vi "TCP Engine.vi"(7 "Hardware Info":T1[](array[typedef]) {"Is Present?" items=["Initializing"=-2, "Unknown"=-1, "Not Present"=0, "Present"=1]}, 8 "error in":errorcluster, 10 "Port":u16=6001, 11 "IP Address":string) -> (0 "error out":errorcluster)   [LabVIEW 2024, in "TCP Engine.lvlib"]
doc: "This VI will communicate with HOST through TCP/IP Communication, also it communicates with all engines through queue mechanism.\n\n\n\nAll Rights Reserved © 2023 SyncSols"
uses:
  TCP Engine.lvlib
  Controls/TCP Engine State Machine Data Cluster.ctl
  Controls/TCP Engine Send Loop Data.ctl
  Main Engine/Controls/Main Engine Command Cluster.ctl
  Main Engine/Controls/Main Engine TCP Command Data.ctl
  Main Engine/Controls/Main Engine Hardware Info Data Cluster.ctl
  Controls/TCP Engine Q Driver Options.ctl
  Controls/TCP Engine State Machine Cases.ctl
  Main Engine/Controls/Main Engine Q Option.ctl
  <vilib>/NI_Real-Time Target Support.lvlib
panel:
  out "notifier":refnum<notifier>
  in  "Data Cluster":T2 {"Hardware Info"."Is Present?" items=["Initializing"=-2, "Unknown"=-1, "Not Present"=0, "Present"=1]}
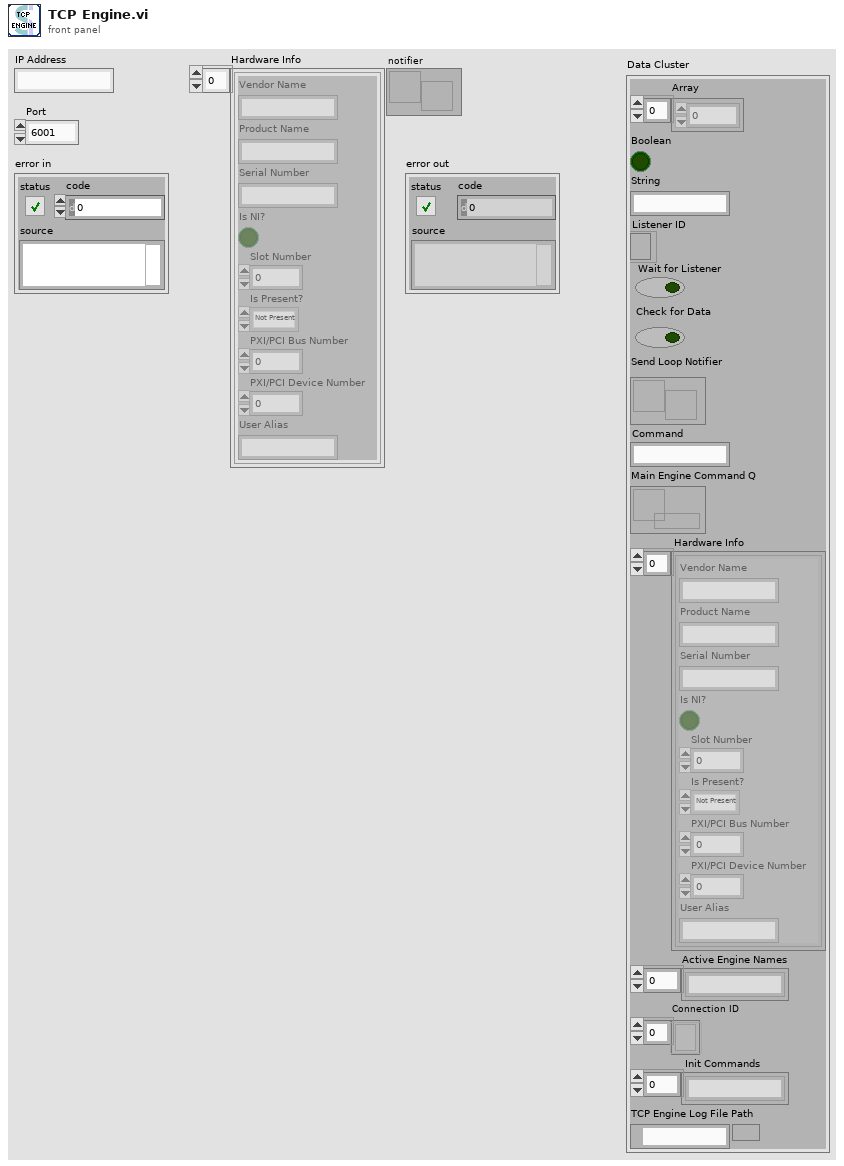
[diagram p1: front panel]
types:
  T1 = typedef "Main Engine Hardware Info Data Cluster.ctl" = cluster{"Vendor Name":string, "Product Name":string, "Serial Number":string, "Is NI?":bool, "Slot Number":i32, "Is Present?":i32, "PXI/PCI Bus Number":u32, "PXI/PCI Device Number":u32, "User Alias":string}
  T2 = typedef "TCP Engine.lvlib/TCP Engine State Machine Data Cluster.ctl" = cluster{"Array":dbl[], "Boolean":bool, "String":string, "Listener ID":refnum<k5>, "Wait for Listener":bool, "Check for Data":bool, "Send Loop Notifier":refnum<notifier>, "Command":string, "Main Engine Command Q":refnum<queue>, "Hardware Info":T1[], "Active Engine Names":string[], "Connection ID":refnum<k5>[], "Init Commands":string[], "TCP Engine Log File Path":path}
  T3 = typedef "TCP Engine.lvlib/TCP Engine Send Loop Data.ctl" = cluster{"Start Send Loop":bool, "Stop Send Loop":bool, "Connection ID":refnum<k5>[], "Log File Path":path}
  T4 = typedef "TCP Engine.lvlib/TCP Engine State Machine Cases.ctl" = enum16{">Poll", ".........State Machine.........", ">Init", ">Init Configuration", ">Decode Configuration", ">Error", ">Exit", "..........TCP Engine..........", ">Wait for Listener", ">Get Msg from HOST", ">Decode the Command", ">Create Listerner ID"}
  T5 = typedef "TCP Engine.lvlib/TCP Engine Q Driver Options.ctl" = enum16{"Initialize", "EnQ", "DeQ", "EnQ at Opp", "Get Q Status", "Flush Q", "Release Q"}
  T6 = typedef "Main Engine Q Option.ctl" = enum16{"Init", "Get"}
  T7 = typedef "Main Engine Command Cluster.ctl" = cluster{"State":T8, "Interface":string, "Engine Name":string, "Varient Data":variant, "SubCmd":string, "Serial Mode":string, "ARINC Board":u8, "Ethernet Mode":u8, "CPU Frequency":dbl}
  T8 = typedef "Main Engine TCP Command Data.ctl" = enum16{"Get HW Info", "Launch Module", "Get CPU Load", "Close CPU Load", "Exit"}
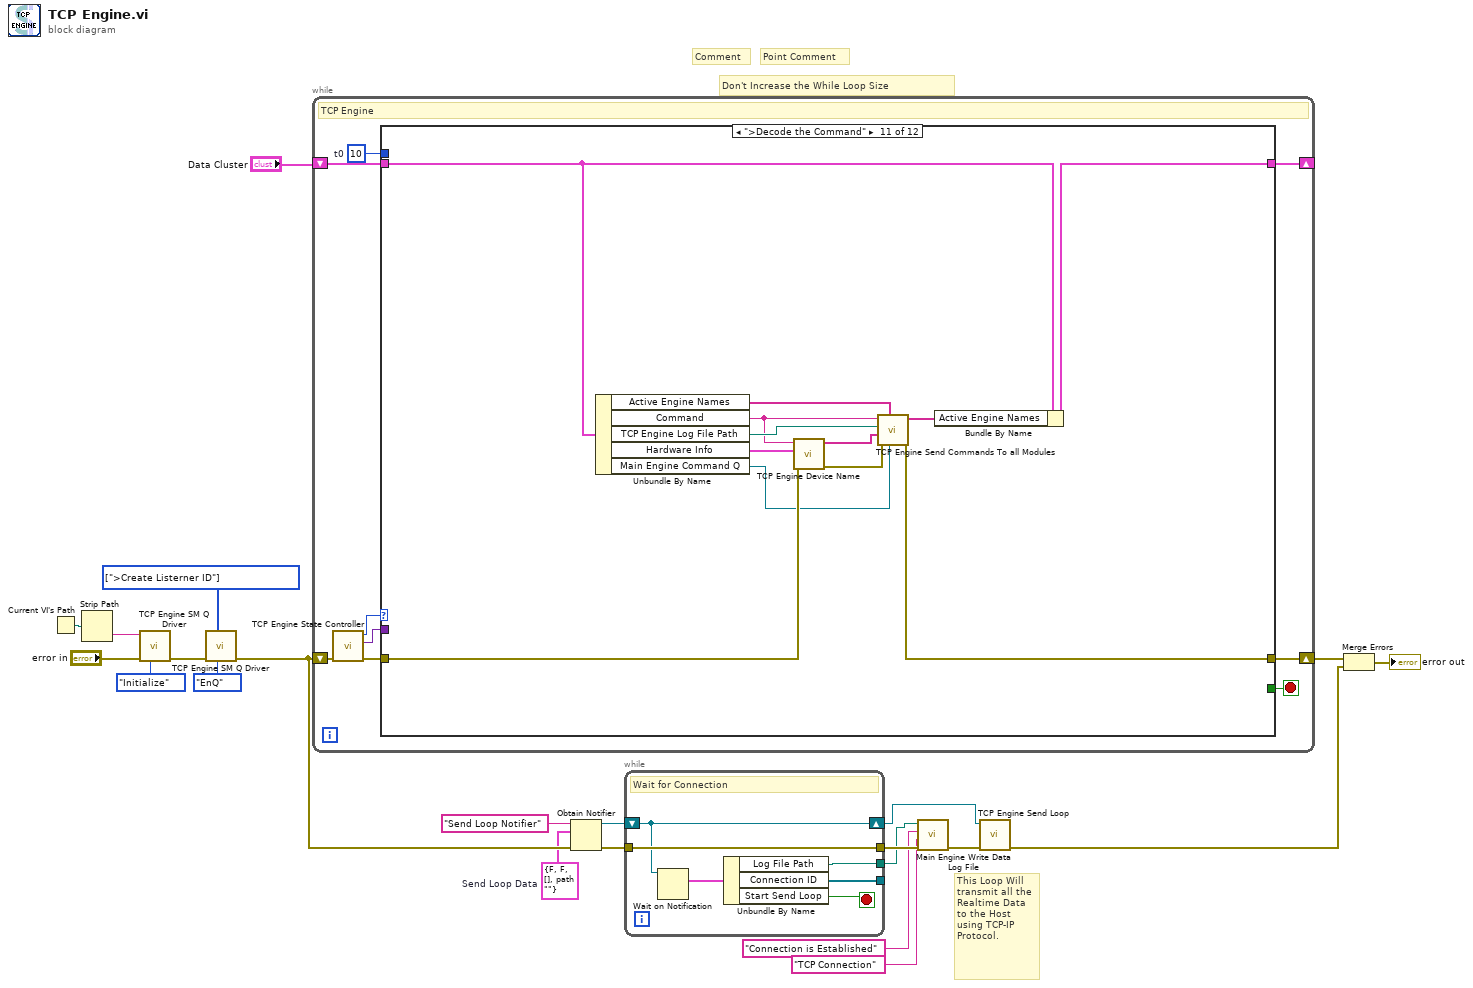
[diagram p0: block diagram]
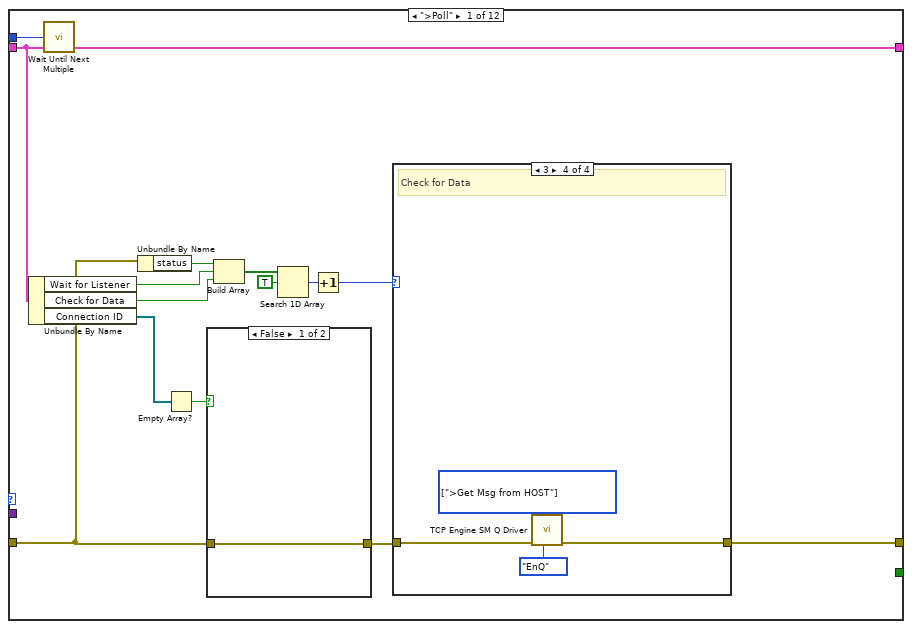
[diagram p2: hidden frame]
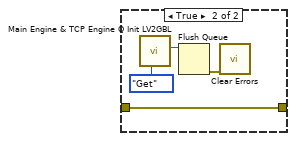
[diagram p3: hidden frame]
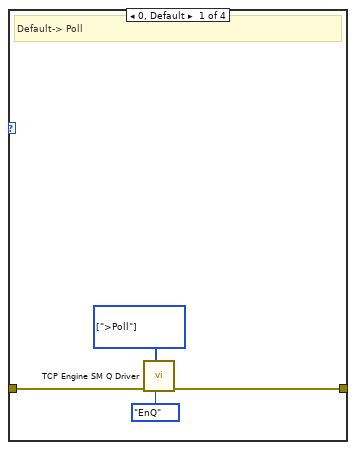
[diagram p4: hidden frame]
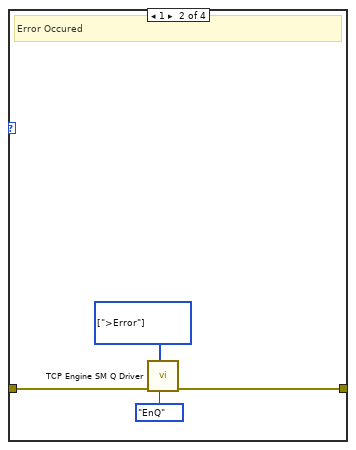
[diagram p5: hidden frame]
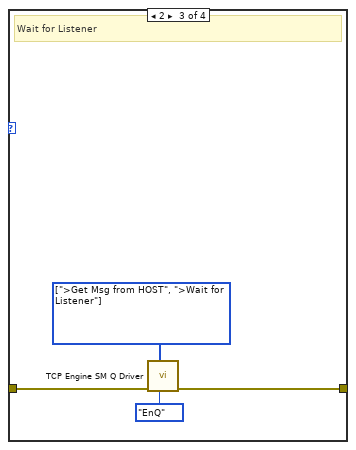
[diagram p6: hidden frame]
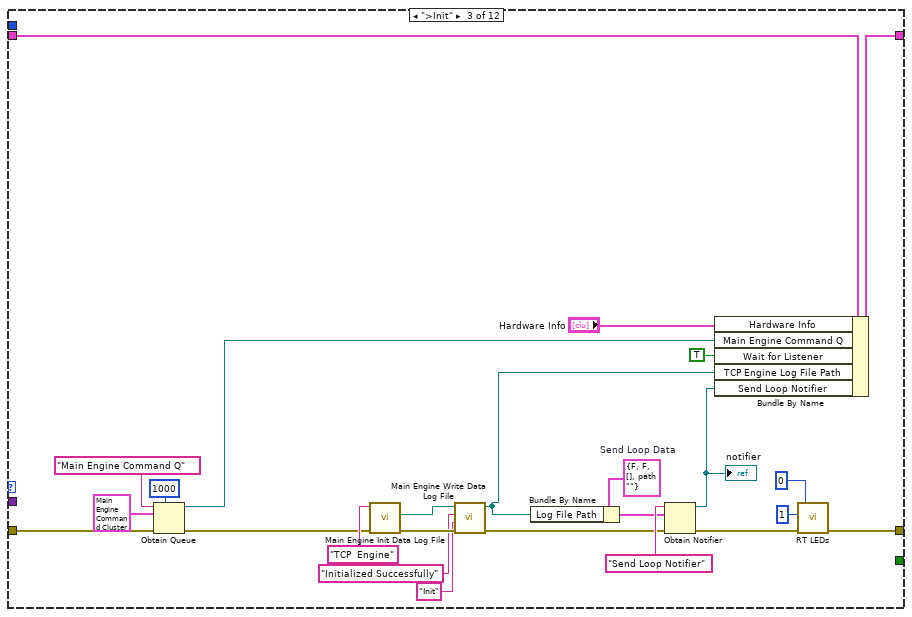
[diagram p8: hidden frame]
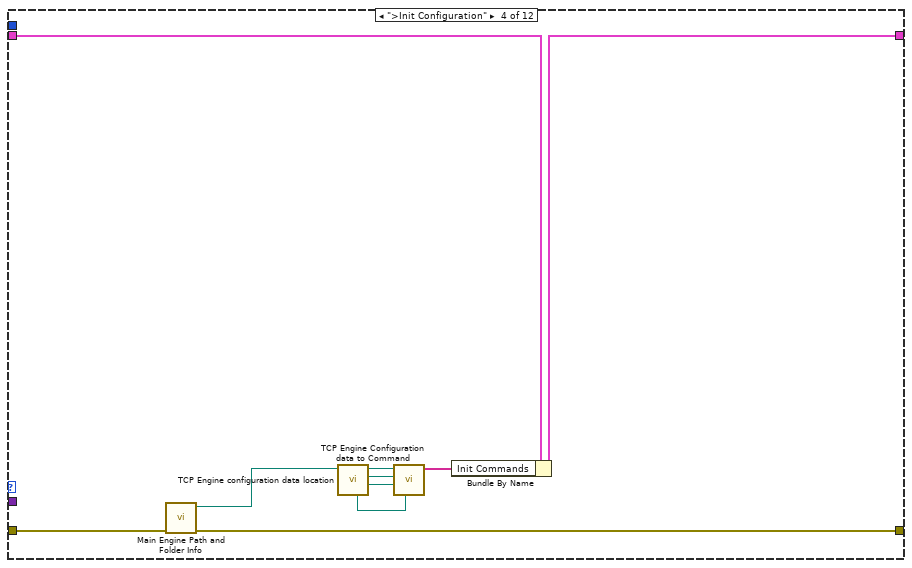
[diagram p9: hidden frame]
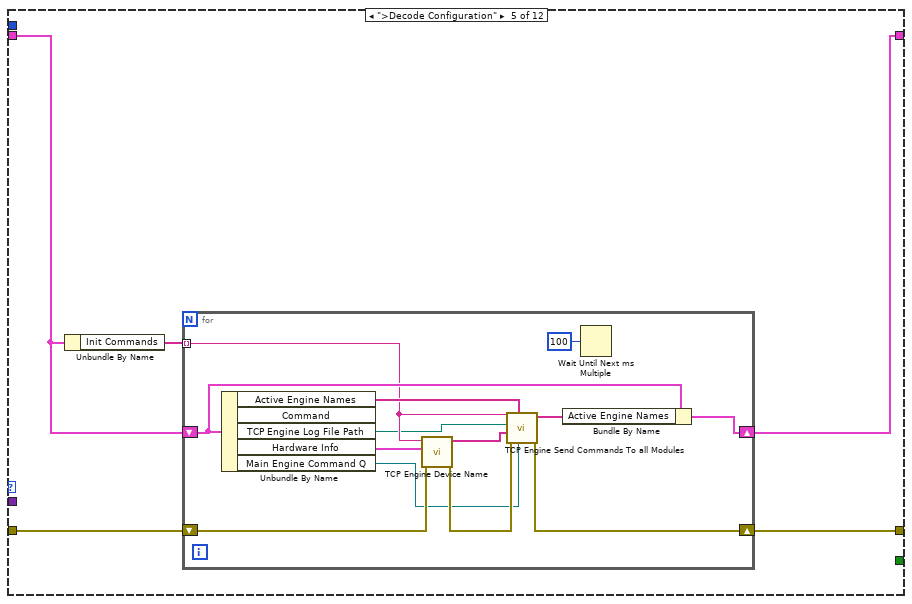
[diagram p10: hidden frame]
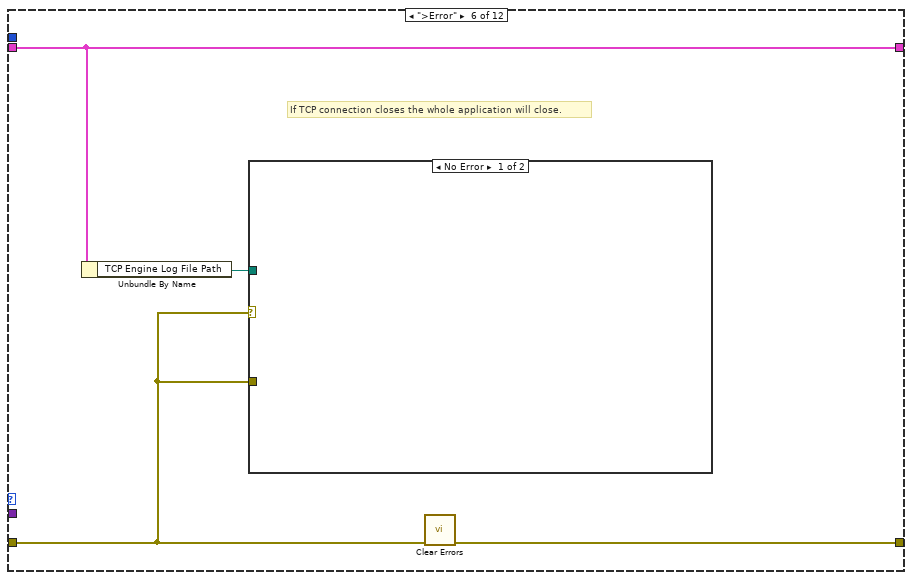
[diagram p11: hidden frame]
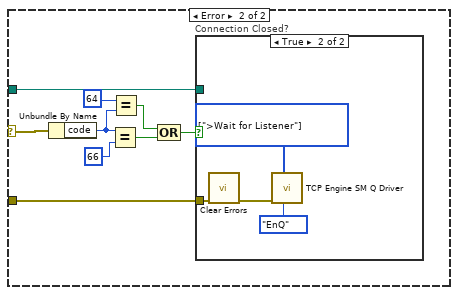
[diagram p12: hidden frame]
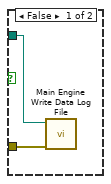
[diagram p13: hidden frame]
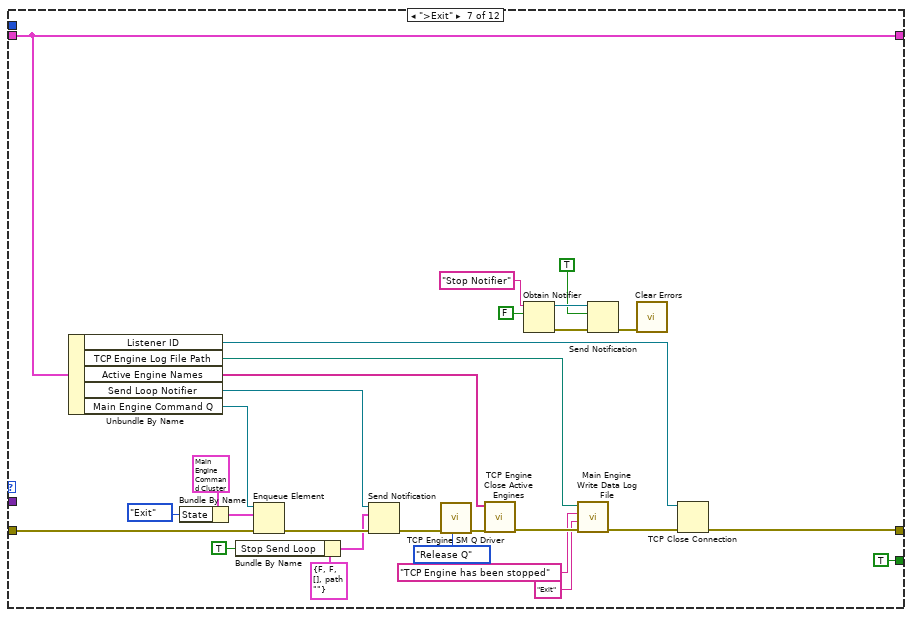
[diagram p14: hidden frame]
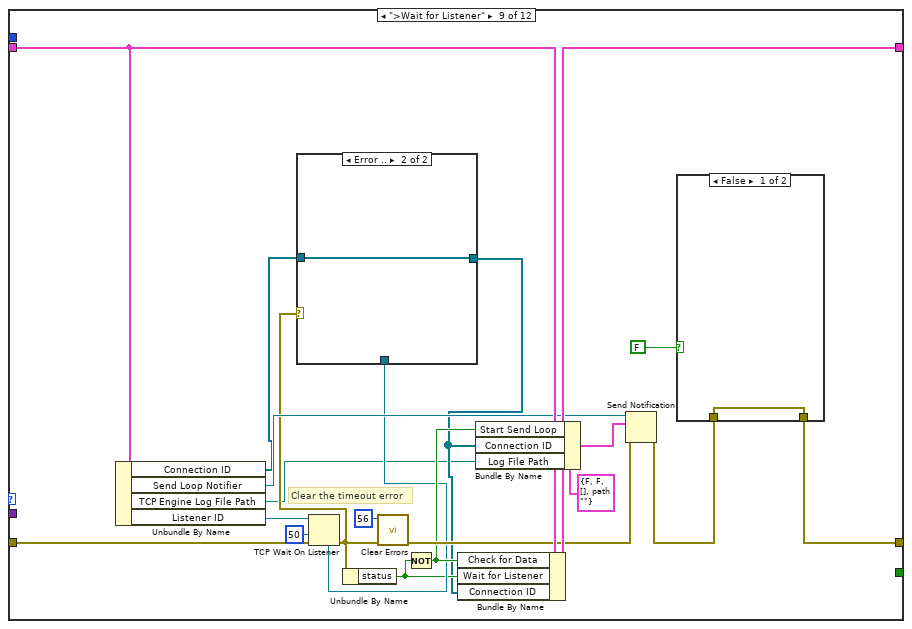
[diagram p16: hidden frame]
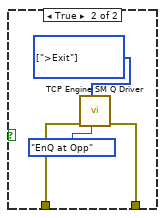
[diagram p17: hidden frame]
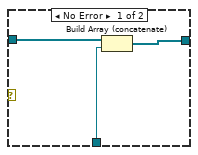
[diagram p18: hidden frame]
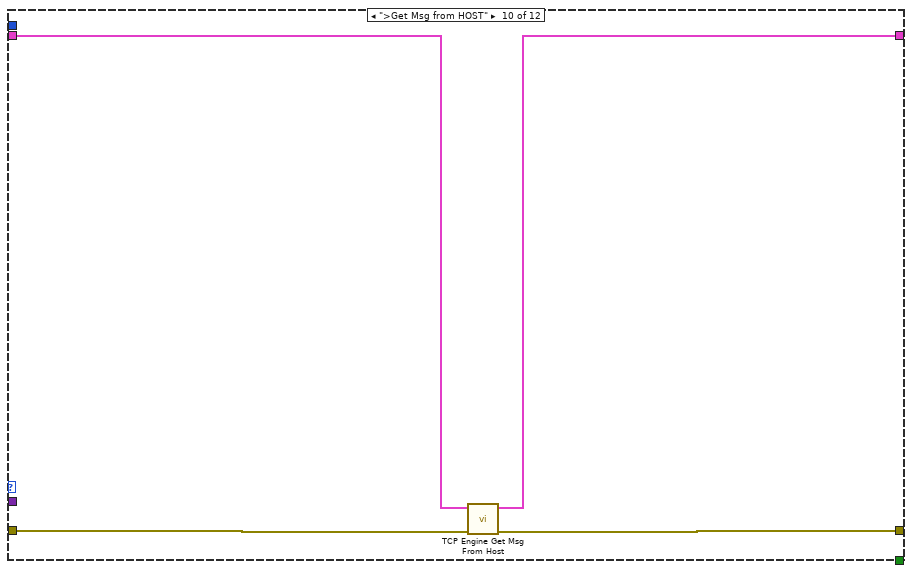
[diagram p19: hidden frame]
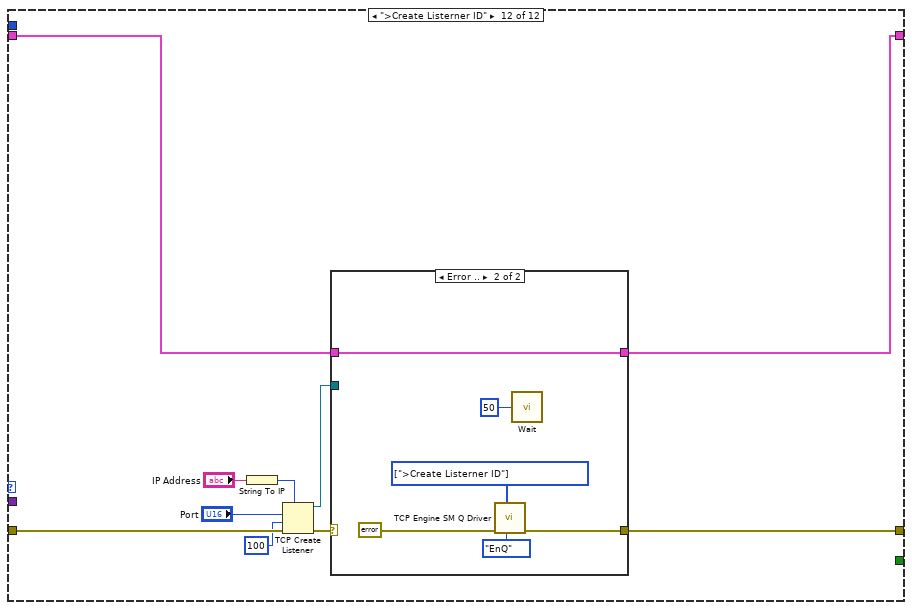
[diagram p20: hidden frame]
diagram:
  w4 = T3 {"Start Send Loop"=FALSE, "Stop Send Loop"=FALSE, "Connection ID"=[], "Log File Path"=path ""}  # Send Loop Data
  w15 = T4[] [enum.">Create Listerner ID"] items=[">Poll", ".........State Machine.........", ">Init", ">Init Configuration", ">Decode Configuration", ">Error", ">Exit", "..........TCP Engine..........", ">Wait for Listener", ">Get Msg from HOST", ">Decode the Command", ">Create Listerner ID"]
  # "This Loop Will transmit all the Realtime Data to the Host using TCP-IP Protocol."
  # "Don't Increase the While Loop Size"
  # "Point Comment"
  # "Comment"
  n1 = Current VI's Path() -> (path=w20:path)
  n2 = Strip Path(path=w20) -> (name=w19:string)  [unwired: 1 out]
  n3 = call "TCP Engine SM Q Driver.vi"("Q Driver Options"=TCP_Engine_Q_Driver_Options."Initialize", "error in"="error in", "Q Name"=w19) -> ("error out"=w17:errorcluster)  [unwired: 4 in, 4 out]
  n4 = call "TCP Engine SM Q Driver.vi"("Q Driver Options"=TCP_Engine_Q_Driver_Options."EnQ", "States"=w15, "error in"=w17) -> ("error out"=w7:errorcluster)  [unwired: 4 in, 4 out]
  n5 = while {
    shift-right: [w31] -> w22
    shift-left: w7 -> [w27]
    shift-right: [w29] -> _
    shift-left: "Data Cluster" -> [w28]
    stop <- w30 stop-if-true
    w23 = u32 10  # t0
    # "TCP Engine"
    n6 = call "TCP Engine State Controller.vi"("error in"=w27) -> ("error out"=w26:errorcluster, "Data"=w24:variant, "SM Cases Options"=w25:T4)  [unwired: 8 in]
    n7 = case shown="\">Decode the Command\"" w25 {
      tunnel: w26 -> [w32 w68 w88 w102 w107 w124 w165 w171 w189 w204 w214 w223]
      tunnel: [w45 w68 w73 w101 w108 w125 w148 w171 w174 w201 w215 w218] -> w31
      tunnel: [_ _ _ _ _ _ TRUE _ _ _ _ _] -> w30
      tunnel: [w39 w67 w93 w95 w106 w123 w167 w170 w187 w202 w209 w219] -> w29
      tunnel: w28 -> [w39 w67 w72 w103 w105 w123 w167 w170 w191 w203 w216 w221]
      tunnel: w24 -> [_ _ _ _ _ _ _ _ _ _ _ _]
      tunnel: w23 -> [w36 _ _ _ _ _ _ _ _ _ _ _]
      frame ">Poll" {
        n8 = Unbundle By Name(w39) -> ("Wait for Listener"=w38:bool, "Check for Data"=w37:bool, "Connection ID"=w35:refnum<k5>[])
        n9 = call "Wait Until Next Multiple"("Count(mSec)"=w36) -> ()  [unwired: 1 out]
        n10 = Unbundle By Name(w32) -> ("status"=w44:bool)
        n11 = Empty Array?(array=w35) -> (empty?=w34:bool)
        n12 = case shown="False" w34 {
          tunnel: [w46 w50] -> w33
          tunnel: w32 -> [w46 w50]
          frame False {
          }
          frame True {
            n13 = call "Main Engine & TCP Engine Q Init LV2GBL.vi"("Q Option"=Main_Engine_Q_Option."Get") -> ("TCP Enigine Tx-Q"=w48:refnum<queue>)  [unwired: 8 in, 2 out]
            n14 = Flush Queue(queue=w48) -> (error out=w47:errorcluster)  [unwired: 1 in, 2 out]
            n15 = call <vilib>:"Clear Errors.vi"("error in (no error)"=w47) -> ()  [unwired: 5 in, 2 out]
          }
        }
        n16 = Build Array(w44, w38, w37) -> (w43:bool[])
        n17 = Search 1D Array(1D array=w43, element=TRUE) -> (index of element=w41:i32)  [unwired: 1 in]
        n18 = Increment(x=w41) -> (x+1=w40:i32)
        n19 = case shown="3" w40 {
          tunnel: w33 -> [w52 w56 w60 w64]
          tunnel: [w51 w55 w59 w63] -> w45
          frame 0, Default {
            w54 = T4[] [enum.">Poll"] items=[">Poll", ".........State Machine.........", ">Init", ">Init Configuration", ">Decode Configuration", ">Error", ">Exit", "..........TCP Engine..........", ">Wait for Listener", ">Get Msg from HOST", ">Decode the Command", ">Create Listerner ID"]
            # "Default-> Poll"
            n20 = call "TCP Engine SM Q Driver.vi"("Q Driver Options"=TCP_Engine_Q_Driver_Options."EnQ", "States"=w54, "error in"=w52) -> ("error out"=w51:errorcluster)  [unwired: 4 in, 4 out]
          }
          frame 1 {
            w57 = T4[] [enum.">Error"] items=[">Poll", ".........State Machine.........", ">Init", ">Init Configuration", ">Decode Configuration", ">Error", ">Exit", "..........TCP Engine..........", ">Wait for Listener", ">Get Msg from HOST", ">Decode the Command", ">Create Listerner ID"]
            # "Error Occured"
            n21 = call "TCP Engine SM Q Driver.vi"("Q Driver Options"=TCP_Engine_Q_Driver_Options."EnQ", "States"=w57, "error in"=w56) -> ("error out"=w55:errorcluster)  [unwired: 4 in, 4 out]
          }
          frame 2 {
            w61 = T4[] [enum.">Get Msg from HOST", enum.">Wait for Listener"] items=[">Poll", ".........State Machine.........", ">Init", ">Init Configuration", ">Decode Configuration", ">Error", ">Exit", "..........TCP Engine..........", ">Wait for Listener", ">Get Msg from HOST", ">Decode the Command", ">Create Listerner ID"]
            # "Wait for Listener"
            n22 = call "TCP Engine SM Q Driver.vi"("Q Driver Options"=TCP_Engine_Q_Driver_Options."EnQ", "States"=w61, "error in"=w60) -> ("error out"=w59:errorcluster)  [unwired: 4 in, 4 out]
          }
          frame 3 {
            w65 = T4[] [enum.">Get Msg from HOST"] items=[">Poll", ".........State Machine.........", ">Init", ">Init Configuration", ">Decode Configuration", ">Error", ">Exit", "..........TCP Engine..........", ">Wait for Listener", ">Get Msg from HOST", ">Decode the Command", ">Create Listerner ID"]
            # "Check for Data"
            n23 = call "TCP Engine SM Q Driver.vi"("Q Driver Options"=TCP_Engine_Q_Driver_Options."EnQ", "States"=w65, "error in"=w64) -> ("error out"=w63:errorcluster)  [unwired: 4 in, 4 out]
          }
        }
      }
      frame ".........State Machine........." {
      }
      frame ">Init" {
        w80 = T3 {"Start Send Loop"=FALSE, "Stop Send Loop"=FALSE, "Connection ID"=[], "Log File Path"=path ""}  # Send Loop Data
        n24 = Obtain Queue(max queue size (-1, unlimited)=1000, name (unnamed)="Main Engine Command Q", element data type=T7 {"State"=enum."Launch Module", "Interface"="AO", "Engine Name"="Slot5_6551_AO", "Varient Data"=variant(string "{"), "SubCmd"="", "Serial Mode"="", "ARINC Board"=0, "Ethernet Mode"=0, "CPU Frequency"=0.0}, error in (no error)=w88) -> (queue out=w86:refnum<queue>, error out=w71:errorcluster)  [unwired: 1 in, 1 out]
        n25 = call "Main Engine Init Data Log File.vi"("error in"=w71, "Engine Name"="TCP  Engine") -> ("error out"=w83:errorcluster, "Log File Path"=w70:path)  [unwired: 8 in]
        n26 = call "Main Engine Write Data Log File.vi"("error in"=w83, "State"="Init", "Input Data"="Initialized Successfully" ("State"), "Log file path In"=w70) -> ("error out"=w79:errorcluster, "Log File Path Out"=w69:path)  [unwired: 6 in]
        n27 = Bundle By Name(cluster=w80, "Log File Path"=w69) -> (w78:T3)
        n28 = Obtain Notifier(name (unnamed)="Send Loop Notifier", notification data type=w78, error in (no error)=w79) -> (notifier out=w77:refnum<notifier>, error out=w74:errorcluster)  [unwired: 1 in, 1 out]
        "notifier" <- w77
        n29 = Bundle By Name(cluster=w72, "Hardware Info"="Hardware Info", "Main Engine Command Q"=w86, "Wait for Listener"=TRUE, "TCP Engine Log File Path"=w69, "Send Loop Notifier"=w77) -> (w93:T2)
        n30 = call <vilib>:"RT LEDs.vi"("error in (no error)"=w74, "State"=1, "LED Num"=0) -> ("error out"=w73:errorcluster)  [unwired: 3 in, 1 out]
      }
      frame ">Init Configuration" {
        n31 = call "Main Engine Path and Folder Info.vi"("error in"=w102) -> ("error out"=w101:errorcluster, "Config"=w100:path)  [unwired: 4 in, 5 out]
        n32 = call "TCP Engine configuration data location.vi"("Directory"=w100) -> ("Serial"=w97:path, "DI"=w98:path, "DO"=w99:path, "AI"=w96:path)  [unwired: 7 in]
        n33 = call "TCP Engine Configuration data to Command.vi"("AI"=w96, "Serial"=w97, "DI"=w98, "DO"=w99) -> ("Command Data"=w94:string[])  [unwired: 7 in]
        n34 = Bundle By Name(cluster=w103, "Init Commands"=w94) -> (w95:T2)
      }
      frame ">Decode Configuration" {
        n35 = Unbundle By Name(w105) -> ("Init Commands"=w104:string[])
        n36 = for {
          shift-right: [w121] -> w108
          shift-left: w107 -> [w120]
          tunnel: w104 -> [w111] mode=indexing
          shift-right: [w115] -> w106
          shift-left: w105 -> [w112]
          n37 = Unbundle By Name(w112) -> ("Active Engine Names"=w113:string[], "TCP Engine Log File Path"=w109:path, "Hardware Info"=w118:T1[], "Main Engine Command Q"=w116:refnum<queue>)  [unwired: 1 out]
          n38 = call "TCP Engine Device Name.vi"("error in"=w120, "Hardware Info"=w118, "JSON String"=w111) -> ("error out"=w119:errorcluster, "Engine Name"=w117:string[])  [unwired: 7 in]
          n39 = call "TCP Engine Send Commands To all Modules.vi"("Main Engine Command Q"=w116, "Active Engine Names"=w113, "error in"=w119, "Engine Name"=w117, "TCP Engine Log File Path"=w109, "JSON String"=w111) -> ("error out"=w121:errorcluster, "Active Engine Names Out"=w114:string[])  [unwired: 4 in]
          n40 = Bundle By Name(cluster=w112, "Active Engine Names"=w114) -> (w115:T2)
          n41 = Wait Until Next ms Multiple(millisecond multiple=u32 100) -> ()  [unwired: 1 out]
        }
      }
      frame ">Error" {
        # "If TCP connection closes the whole application will close."
        n42 = Unbundle By Name(w123) -> ("TCP Engine Log File Path"=w122:path)
        n43 = case shown="No Error" w124 {
          selector: w124 -> [_ w134]
          tunnel: w124 -> [_ w132]
          tunnel: w122 -> [_ w126]
          frame No Error {
          }
          frame Error {
            n44 = Unbundle By Name(w134) -> ("code"=w130:i32)
            n45 = Equal?(x=w130, y=66) -> (x = y?=w127:bool)
            n46 = Equal?(x=64 ("y"), y=w130) -> (x = y?=w128:bool)
            n47 = Compound Arithmetic op=OR(w128, w127) -> (w129:bool)
            n48 = case "Connection Closed?" shown="True" w129 {
              tunnel: w132 -> [w136 w137]
              tunnel: w126 -> [w135 _]
              frame False {
                n49 = call "Main Engine Write Data Log File.vi"("error in"=w136, "Log file path In"=w135) -> ()  [unwired: 8 in, 2 out]
              }
              frame True {
                w139 = T4[] [enum.">Wait for Listener"] items=[">Poll", ".........State Machine.........", ">Init", ">Init Configuration", ">Decode Configuration", ">Error", ">Exit", "..........TCP Engine..........", ">Wait for Listener", ">Get Msg from HOST", ">Decode the Command", ">Create Listerner ID"] ("States")
                n50 = call <vilib>:"Clear Errors.vi"("error in (no error)"=w137) -> ("error out"=w138:errorcluster)  [unwired: 5 in, 1 out]
                n51 = call "TCP Engine SM Q Driver.vi"("Q Driver Options"=TCP_Engine_Q_Driver_Options."EnQ", "States"=w139, "error in"=w138) -> ()  [unwired: 4 in, 5 out]
              }
            }
          }
        }
        n52 = call <vilib>:"Clear Errors.vi"("error in (no error)"=w124) -> ("error out"=w125:errorcluster)  [unwired: 5 in, 1 out]
      }
      frame ">Exit" {
        n53 = Unbundle By Name(w167) -> ("Listener ID"=w149:refnum<k5>, "TCP Engine Log File Path"=w141:path, "Active Engine Names"=w154:string[], "Send Loop Notifier"=w164:refnum<notifier>, "Main Engine Command Q"=w166:refnum<queue>)
        n54 = Bundle By Name(cluster=T7 {"State"=enum."Launch Module", "Interface"="AO", "Engine Name"="Slot5_6551_AO", "Varient Data"=variant(string "{"), "SubCmd"="", "Serial Mode"="", "ARINC Board"=0, "Ethernet Mode"=0, "CPU Frequency"=0.0} ("element"), "State"=Main_Engine_TCP_Command_Data."Exit" ("element")) -> (w156:T7)
        n55 = Bundle By Name(cluster=T3 {"Start Send Loop"=FALSE, "Stop Send Loop"=FALSE, "Connection ID"=[], "Log File Path"=path ""} ("notification"), "Stop Send Loop"=TRUE) -> (w160:T3)
        n56 = Enqueue Element(queue=w166, element=w156, error in (no error)=w165) -> (error out=w163:errorcluster)  [unwired: 1 in, 2 out]
        n57 = Send Notification(notification=w160, notifier=w164, error in (no error)=w163) -> (error out=w162:errorcluster)  [unwired: 1 out]
        n58 = call "TCP Engine SM Q Driver.vi"("Q Driver Options"=TCP_Engine_Q_Driver_Options."Release Q", "error in"=w162) -> ("error out"=w155:errorcluster)  [unwired: 5 in, 4 out]
        n59 = call "TCP Engine Close Active Engines.vi"("error in"=w155, "Engines Name"=w154) -> ("error out"=w153:errorcluster)  [unwired: 9 in]
        n60 = Obtain Notifier(name (unnamed)="Stop Notifier", notification data type=FALSE) -> (notifier out=w144:refnum<notifier>, error out=w145:errorcluster)  [unwired: 2 in, 1 out]
        n61 = call "Main Engine Write Data Log File.vi"("error in"=w153, "State"="Exit" ("Input Data"), "Input Data"="TCP Engine has been stopped", "Log file path In"=w141) -> ("error out"=w152:errorcluster)  [unwired: 6 in, 1 out]
        n62 = Send Notification(notification=TRUE, notifier=w144, error in (no error)=w145) -> (error out=w142:errorcluster)  [unwired: 1 out]
        n63 = call <vilib>:"Clear Errors.vi"("error in (no error)"=w142) -> ()  [unwired: 5 in, 2 out]
        n64 = TCP Close Connection(connection ID=w149, error in (no error)=w152) -> (error out=w148:errorcluster)  [unwired: 1 in, 1 out]
      }
      frame "..........TCP Engine.........." {
      }
      frame ">Wait for Listener" {
        # "Clear the timeout error"
        n65 = Unbundle By Name(w191) -> ("Connection ID"=w180:refnum<k5>[], "Send Loop Notifier"=w184:refnum<notifier>, "TCP Engine Log File Path"=w172:path, "Listener ID"=w190:refnum<k5>)
        n66 = TCP Wait On Listener(8:w189, 9:50 ("timeout ms (wait forever: -1)"), 11:w190) -> (0:w179:errorcluster, 4:w178:refnum<k5>)  [unwired: 1 in, 3 out]
        n67 = case shown="Error .." w179 {
          tunnel: w180 -> [w199 w200]
          tunnel: w178 -> [w198 _]
          tunnel: [w197 w200] -> w176
          frame No Error {
            n68 = Build Array (concatenate)(w199, w198) -> (w197:refnum<k5>[])
          }
          frame Error {
          }
        }
        n69 = Unbundle By Name(w179) -> ("status"=w177:bool)
        n70 = call <vilib>:"Clear Errors.vi"("error in (no error)"=w179, "specific error code to clear (0: all)"=56) -> ("error out"=w185:errorcluster)  [unwired: 4 in, 1 out]
        n71 = Not(x=w177) -> (.not. x?=w181:bool)
        n72 = Bundle By Name(cluster=w191, "Check for Data"=w181, "Wait for Listener"=w177, "Connection ID"=w176) -> (w187:T2)
        n73 = Bundle By Name(cluster=T3 {"Start Send Loop"=FALSE, "Stop Send Loop"=FALSE, "Connection ID"=[], "Log File Path"=path ""} ("notification"), "Start Send Loop"=w181, "Connection ID"=w176, "Log File Path"=w172) -> (w182:T3)
        n74 = Send Notification(notification=w182, notifier=w184, error in (no error)=w185) -> (error out=w175:errorcluster)  [unwired: 1 out]
        n75 = case shown="False" FALSE {
          tunnel: w175 -> [w192 w194]
          tunnel: [w192 w193] -> w174
          frame False {
          }
          frame True {
            w195 = T4[] [enum.">Exit"] items=[">Poll", ".........State Machine.........", ">Init", ">Init Configuration", ">Decode Configuration", ">Error", ">Exit", "..........TCP Engine..........", ">Wait for Listener", ">Get Msg from HOST", ">Decode the Command", ">Create Listerner ID"]
            n76 = call "TCP Engine SM Q Driver.vi"("Q Driver Options"=TCP_Engine_Q_Driver_Options."EnQ at Opp", "States"=w195, "error in"=w194) -> ("error out"=w193:errorcluster)  [unwired: 4 in, 4 out]
          }
        }
      }
      frame ">Get Msg from HOST" {
        n77 = call "TCP Engine Get Msg From Host.vi"("error in (no error)"=w204, "Data Cluster in"=w203) -> ("error out"=w201:errorcluster, "Data Cluster out"=w202:T2)  [unwired: 8 in]
      }
      frame ">Decode the Command" {
        n78 = Unbundle By Name(w216) -> ("Active Engine Names"=w207:string[], "Command"=w205:string, "TCP Engine Log File Path"=w206:path, "Hardware Info"=w212:T1[], "Main Engine Command Q"=w210:refnum<queue>)
        n79 = call "TCP Engine Device Name.vi"("error in"=w214, "Hardware Info"=w212, "JSON String"=w205) -> ("error out"=w213:errorcluster, "Engine Name"=w211:string[])  [unwired: 7 in]
        n80 = call "TCP Engine Send Commands To all Modules.vi"("Main Engine Command Q"=w210, "Active Engine Names"=w207, "error in"=w213, "Engine Name"=w211, "TCP Engine Log File Path"=w206, "JSON String"=w205) -> ("error out"=w215:errorcluster, "Active Engine Names Out"=w208:string[])  [unwired: 4 in]
        n81 = Bundle By Name(cluster=w216, "Active Engine Names"=w208) -> (w209:T2)
      }
      frame ">Create Listerner ID" {
        n82 = String To IP(1:"IP Address") -> (0:w225:u32)
        n83 = TCP Create Listener(7:w225, 8:w223, 9:100 ("timeout ms (25000)"), 10:"Port") -> (0:w222:errorcluster, 3:w220:refnum<k5>)  [unwired: 1 in, 1 out]
        n84 = case shown="Error .." w222 {
          selector: w222 -> [w228 _]
          tunnel: w221 -> [w233 w239]
          tunnel: w220 -> [w232 _]
          tunnel: [w231 w239] -> w219
          tunnel: [w227 w235] -> w218
          frame No Error {
            w230 = T4[] [enum.">Init", enum.">Init Configuration", enum.">Decode Configuration"] items=[">Poll", ".........State Machine.........", ">Init", ">Init Configuration", ">Decode Configuration", ">Error", ">Exit", "..........TCP Engine..........", ">Wait for Listener", ">Get Msg from HOST", ">Decode the Command", ">Create Listerner ID"]
            n85 = Bundle By Name(cluster=w233, "Listener ID"=w232) -> (w231:T2)
            n86 = call "TCP Engine SM Q Driver.vi"("Q Driver Options"=TCP_Engine_Q_Driver_Options."EnQ", "States"=w230, "error in"=w228) -> ("error out"=w227:errorcluster)  [unwired: 4 in, 4 out]
          }
          frame Error {
            w238 = T4[] [enum.">Create Listerner ID"] items=[">Poll", ".........State Machine.........", ">Init", ">Init Configuration", ">Decode Configuration", ">Error", ">Exit", "..........TCP Engine..........", ">Wait for Listener", ">Get Msg from HOST", ">Decode the Command", ">Create Listerner ID"]
            n87 = call "TCP Engine SM Q Driver.vi"("Q Driver Options"=TCP_Engine_Q_Driver_Options."EnQ", "States"=w238, "error in"=errorcluster {"status"=FALSE, "code"=0, "source"=""}) -> ("error out"=w235:errorcluster)  [unwired: 4 in, 4 out]
            n88 = call "Wait"("Count(mSec)"=u32 50) -> ()  [unwired: 1 out]
          }
        }
      }
    }
  }
  n89 = Obtain Notifier(name (unnamed)="Send Loop Notifier", notification data type=w4, error in (no error)=w7) -> (notifier out=w5:refnum<notifier>, error out=w3:errorcluster)  [unwired: 1 in, 1 out]
  n90 = while {
    tunnel: w3 -> [w242]
    tunnel: [w243] -> _
    tunnel: [w242] -> w11
    tunnel: [w240] -> w1
    shift-right: [w241] -> w14
    shift-left: w5 -> [w241]
    stop <- w244 stop-if-true
    # "Wait for Connection"
    n91 = Wait on Notification(notifier=w241) -> (notification=w245:T3)  [unwired: 3 in, 3 out]
    n92 = Unbundle By Name(w245) -> ("Log File Path"=w240:path, "Connection ID"=w243:refnum<k5>[], "Start Send Loop"=w244:bool)
  }
  n93 = call "Main Engine Write Data Log File.vi"("error in"=w11, "State"="TCP Connection", "Input Data"="Connection is Established" ("State"), "Log file path In"=w1) -> ("error out"=w10:errorcluster)  [unwired: 6 in, 1 out]
  n94 = call "TCP Engine Send Loop.vi"("error in (no error)"=w10, "Send Loop Notifier"=w14) -> ("error out"=w12:errorcluster)  [unwired: 9 in]
  n95 = Merge Errors(w22, w12) -> (→"error out":errorcluster)
